vi "Image format and conditioning.vi"(9 "Peak value in dataset (I16)":dbl=32767.0, 10 "Intensity":dbl, 11 "Image Array(Single Trial)":i16[][](array[numeric])) -> (3 "Array":u8[][](array[numeric]))   [LabVIEW 2020]
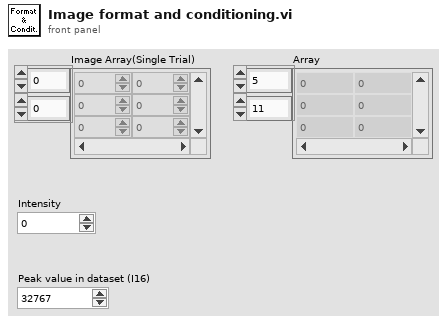
[diagram p1: front panel]
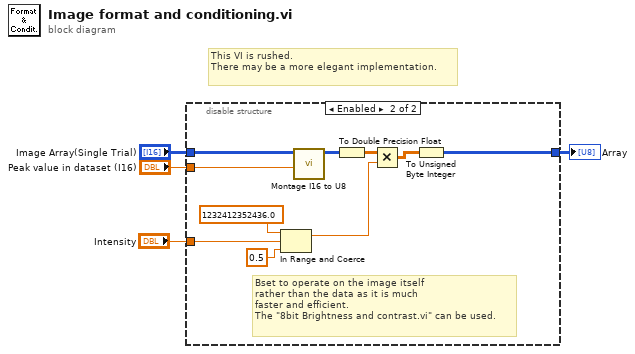
[diagram p0: block diagram]
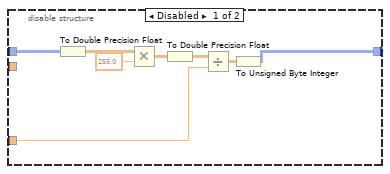
[diagram p2: hidden frame]
diagram:
  # "This VI is rushed.\nThere may be a more elegant implementation."
  n1 = disable-structure shown="Enabled" {
    disable-tunnel: "Intensity" -> [w12 w16]
    disable-tunnel: "Image Array(Single Trial)" -> [w10 w22]
    disable-tunnel: [w6 w18] -> w2
    disable-tunnel: "Peak value in dataset (I16)" -> [_ w13]
    frame Disabled {
      n2 = To Double Precision Float(number=w10) -> (double precision float=w5:dbl[][])
      n3 = Multiply(x=w5, y=255.0 ("Number of frames")) -> (x*y=w7:dbl[][])
      n4 = To Double Precision Float(number=w7) -> (double precision float=w8:dbl[][])
      n5 = Divide(x=w8, y=w12) -> (x/y=w11:dbl[][])
      n6 = To Unsigned Byte Integer(number=w11) -> (unsigned 8bit integer=w6:u8[][])
    }
    frame Enabled {
      # "Bset to operate on the image itself\nrather than the data as it is much \nfaster and efficient.\nThe \"8bit Brightness and contrast.vi\" can be used."
      n7 = In Range and Coerce(upper limit=1232412352436.0, x=w16, lower limit=0.5) -> (coerced(x)=w15:dbl)  [unwired: 1 out]
      n8 = call "Montage I16 to U8.vi"("Maximum intensity in I16 data"=w13, "I16 (positive only / 0-32767)"=w22) -> ("U8 (0-255)"=w21:u8[][])  [unwired: 9 in]
      n9 = To Double Precision Float(number=w21) -> (double precision float=w19:dbl[][])
      n10 = Multiply(x=w19, y=w15) -> (x*y=w20:dbl[][])
      n11 = To Unsigned Byte Integer(number=w20) -> (unsigned 8bit integer=w18:u8[][])
    }
  }
  "Array" <- w2
